vi "Auto_template.vi"() -> ()   [LabVIEW 2012]
uses:
  <vilib>/NXT/Subs/LVHSConnector.ctl
  <vilib>/NXT/LegoClasses/BrickReference/BrickReference.lvclass
  <vilib>/NXT/Block Support/NXT_ButtonSelector.ctl
  <vilib>/NXT/Dual Mode Library/Display/drawText.vi
  <vilib>/NXT/Dual Mode Library/Waits/Wait_Num(msec).vi
  <vilib>/NXT/Dual Mode Library/prims/inRangeAndCoerce/inRangeAndCoerce_int.vi
  <vilib>/NXT/Dual Mode Library/Display/drawNumber.vi
  <vilib>/NXT/Dual Mode Library/Sound/Tone.vi
panel:
  out "Enabled":bool
  out "iter":i32
  out "NXT":T1
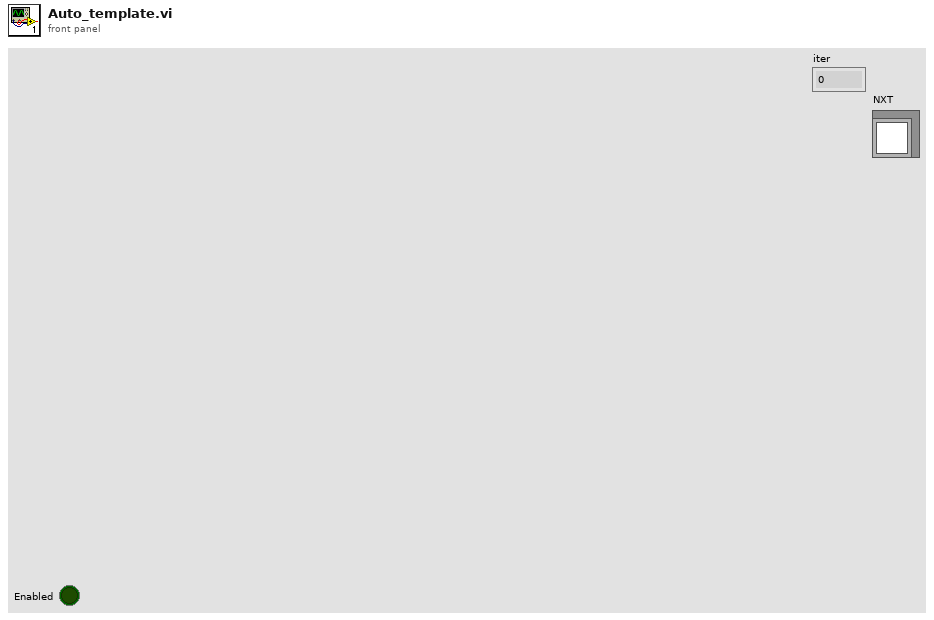
[diagram p1: front panel]
types:
  T1 = typedef "LVHSConnector.ctl" = refnum<class "BrickReference.lvclass">
  T2 = typedef "NXT_ButtonSelector.ctl" = u16
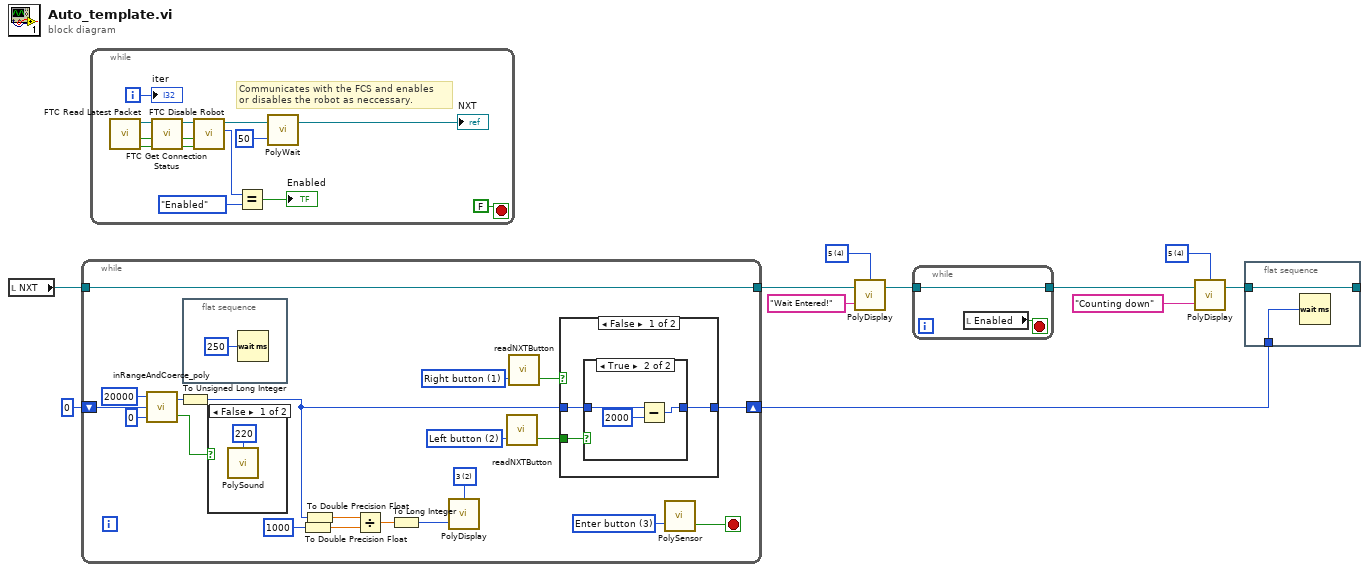
[diagram p0: block diagram]
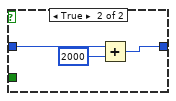
[diagram p4: hidden frame]
diagram:
  w6 = i16 4 items=["1", "2", "3", "4", "5", "6", "7", "8"] ("Line")
  w7 = i16 4 items=["1", "2", "3", "4", "5", "6", "7", "8"] ("Line")
  n1 = local read "NXT"() -> (w1:T1)
  n2 = while {
    tunnel: [w31] -> w9
    tunnel: w1 -> [w31]
    shift-right: [w24] -> w10
    shift-left: u32 0 ("Power/Speed 1") -> [w17]
    stop <- w29 stop-if-true
    w23 = i16 2 items=["1", "2", "3", "4", "5", "6", "7", "8"] ("Line")
    w26 = T2 1 items=["Enter button"=3, "Left button"=2, "Right button"=1] ("Button (Enter button)")
    w25 = T2 2 items=["Enter button"=3, "Left button"=2, "Right button"=1] ("Button (Enter button)")
    w30 = T2 3 items=["Enter button"=3, "Left button"=2, "Right button"=1] ("Button (Enter button)")
    n3 = call-poly <vilib>:"inRangeAndCoerce_poly.vi"("lower limit"=0, "x"=w17, "upper limit"=20000) -> ("In Range?"=w12:bool, "coerced(x)"=w14:i32)
    n4 = To Unsigned Long Integer(number=w14) -> (unsigned 32bit integer=w13:u32)
    n5 = flat-sequence {
      frame #0 {
        n6 = Wait (ms)(milliseconds to wait=u32 250) -> ()  [unwired: 1 out]
      }
    }
    n7 = case shown="False" w12 {
      frame False {
        n8 = call-poly <vilib>:"PolySound.vi"("Tone (440 Hz)"=u16 220) -> ()  [unwired: 3 in, 1 out]
      }
      frame True {
      }
    }
    n9 = To Double Precision Float(number=u32 1000 ("Power/Speed 1")) -> (double precision float=w18:dbl)
    n10 = To Double Precision Float(number=w13) -> (double precision float=w20:dbl)
    n11 = Divide(x=w20, y=w18) -> (x/y=w21:dbl)
    n12 = To Long Integer(number=w21) -> (32bit integer=w19:i32)
    n13 = call-poly <vilib>:"PolyDisplay.vi"("number"=w19, "Line"=w23) -> ()  [unwired: 2 in, 1 out]
    n14 = call <vilib>:"readNXTButton.vi"("Button (Enter button)"=w25) -> ("Yes/No"=w28:bool)  [unwired: 2 in, 1 out]
    n15 = call <vilib>:"readNXTButton.vi"("Button (Enter button)"=w26) -> ("Yes/No"=w27:bool)  [unwired: 2 in, 1 out]
    n16 = case shown="False" w27 {
      tunnel: w28 -> [w36 _]
      tunnel: [w35 w42] -> w24
      tunnel: w13 -> [w34 w43]
      frame False {
        n17 = case shown="True" w36 {
          tunnel: [w37 w39] -> w35
          tunnel: w34 -> [w37 w40]
          frame False {
          }
          frame True {
            n18 = Subtract(x=w40, y=u32 2000) -> (x-y=w39:u32)
          }
        }
      }
      frame True {
        n19 = Add(x=w43, y=u32 2000) -> (x+y=w42:u32)
      }
    }
    n20 = call-poly <vilib>:"PolySensor.vi"("Button (Enter button)"=w30) -> ("Yes/No"=w29:bool)  [unwired: 2 in, 1 out]
  }
  n21 = while {
    i -> [w45]
    stop <- FALSE stop-if-true
    # "Communicates with the FCS and enables \nor disables the robot as neccessary."
    n22 = call <vilib>:"FTC Read Latest Packet.vi"() -> ("Packet Received?"=w55:bool, "Stopped?"=w54:bool, "NXT"=w57:T1)  [unwired: 6 in, 3 out]
    n23 = call <vilib>:"FTC Get Connection Status.vi"("Packet Received?"=w55, "Stopped?"=w54, "NXT"=w57) -> ("Online?"=w47:bool, "Stopped?"=w48:bool, "NXT"=w56:T1)  [unwired: 5 in]
    n24 = call <vilib>:"FTC Disable Robot.vi"("Online?"=w47, "Stopped?"=w48, "NXT"=w56) -> ("Enabled?"=w51:enum16{"Disabled", "Enabled"}, "NXT"=w53:T1)  [unwired: 3 in]
    n25 = Equal?(x=w51, y=enum16{"Disabled", "Enabled"}."Enabled") -> (x = y?=→"Enabled":bool)
    n26 = call-poly <vilib>:"PolyWait.vi"("Time (100 msec)"=u32 50 ("Time (msec)"), "NXT"=w53) -> ("NXT"=→"NXT":T1)  [unwired: 2 in]
    "iter" <- w45
  }
  n27 = call-poly <vilib>:"PolyDisplay.vi"("Text"="Wait Entered!", "NXT"=w9, "Line"=w7) -> ("NXT"=w3:T1)  [unwired: 1 in]
  n28 = while {
    tunnel: [w58] -> w2
    tunnel: w3 -> [w58]
    stop <- w59 stop-if-true
    n29 = local read "Enabled"() -> (w59:bool)
  }
  n30 = call-poly <vilib>:"PolyDisplay.vi"("Text"="Counting down", "NXT"=w2, "Line"=w6) -> ("NXT"=w4:T1)  [unwired: 1 in]
  n31 = flat-sequence {
    tunnel: w4 -> [w61]
    tunnel: [w61] -> _
    tunnel: w10 -> [w60]
    frame #0 {
      n32 = Wait (ms)(milliseconds to wait=w60) -> ()  [unwired: 1 out]
    }
  }
